vi "Process.vi"(8 "error in (no error)":errorcluster, 10 "Pound in":refnum<class "Pound.lvclass">, 11 "Qbus in":refnum<class "Qbus.lvclass">) -> (0 "error out":errorcluster)   [LabVIEW 2017, in "McsaFpgaBitfileManager.lvlib"]
doc: "Downloads the appropriate bitfile to the device FPGA so that the device can begin to acquire data. The FPGA Acquisition process cannot initiate data acquisition until the device FPGA receives the bitfile."
uses:
  <vilib>/addons/InsightCM/Devices/Shared/Mcsa/McsaFpgaBitfileManager/McsaFpgaBitfileManager.lvlib
  <vilib>/addons/Qbus/Qbus.lvclass
  <vilib>/NI/Software Watchdog/Pound/Pound.lvclass
  <vilib>/addons/InsightCM/Devices/Shared/Mcsa/McsaFpgaBitfileManager/controls/config.ctl
  <vilib>/FPGAPlugInAG/Dynamic/niLvFpga_Close_Dynamic.vi
  <vilib>/rvi/interface/nirviCloseFPGA/nirviCloseFPGA.xnode
  <vilib>/NI/Software Watchdog/Watchdog/Watchdog.lvclass
  <vilib>/addons/InsightCM/Devices/Shared/Common/FpgaBitfileManager/FpgaBitfileManager.lvlib
  <vilib>/addons/InsightCM/Utilities/GlobalConfiguration/GlobalConfiguration.lvlib
  <vilib>/addons/TraceLogger/TraceLogger.lvlib
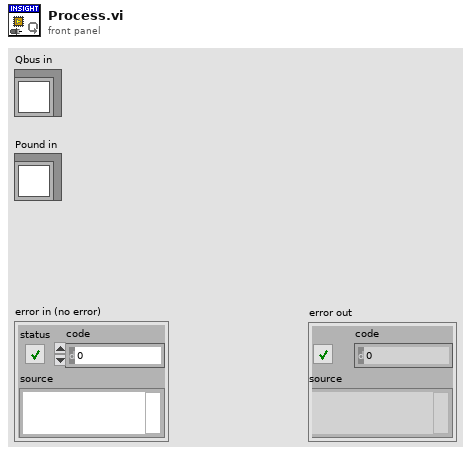
[diagram p1: front panel]
types:
  T1 = typedef "McsaFPGABitfileManager.lvlib/config.ctl" = cluster{"Bitfile reference":refnum<k20>}
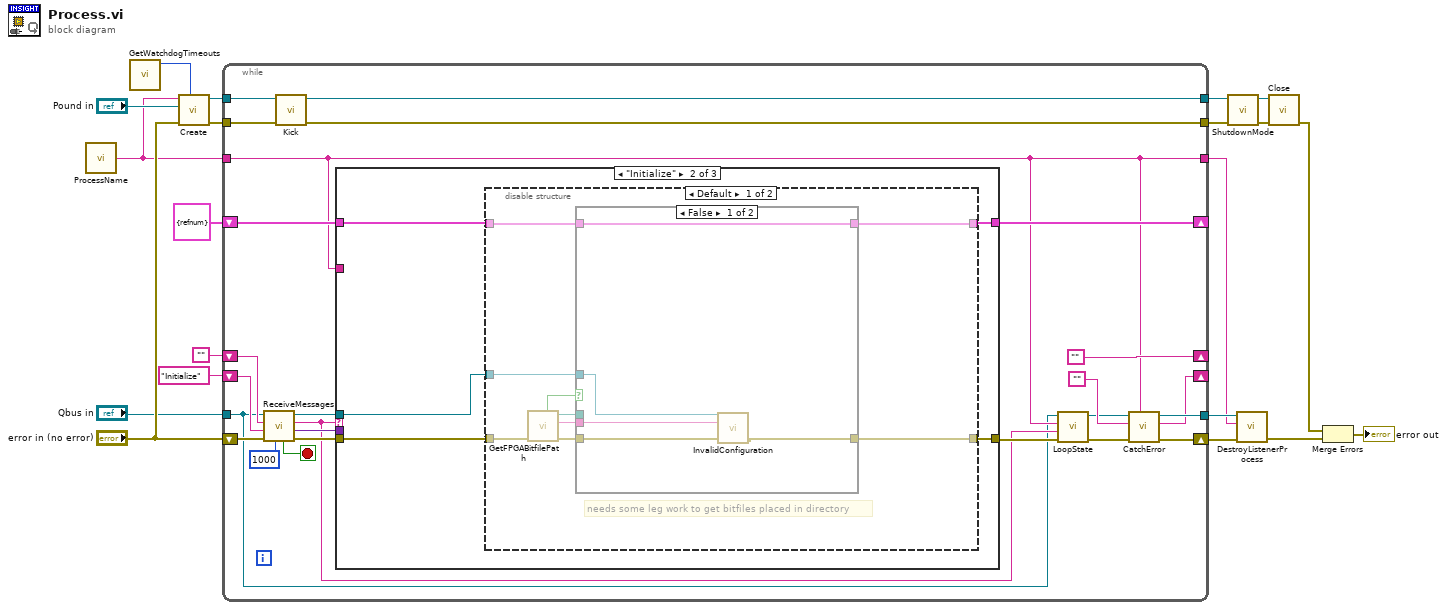
[diagram p0: block diagram]
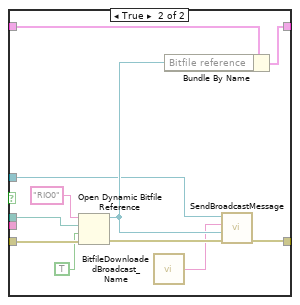
[diagram p3: hidden frame]
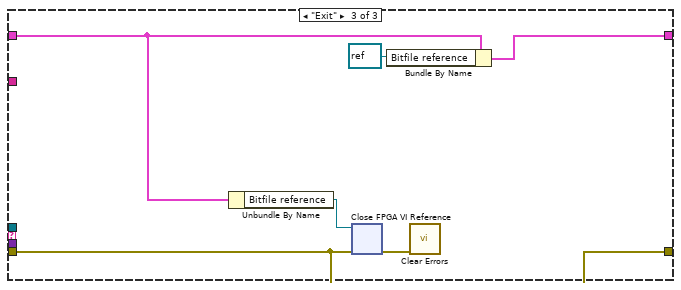
[diagram p5: hidden frame]
diagram:
  n1 = call <vilib>:"ProcessName.vi"() -> ("process name"=w1:string)  [unwired: 5 in]
  n2 = call <vilib>:"GetWatchdogTimeouts.vi"() -> ("software timeout"=w2:u32)  [unwired: 10 in, 1 out]
  n3 = call <vilib>:"Create.vi"("Execution Timeout (ms)"=w2, "error in (no error)"="error in (no error)", "Pound"="Pound in", "Name"=w1) -> ("error out"=w9:errorcluster, "Watchdog"=w14:refnum<data-value>)  [unwired: 6 in]
  n4 = while {
    shift-right: [""] -> _
    shift-left: "" -> [w44]
    tunnel: "Qbus in" -> [w24]
    tunnel: w1 -> [w31]
    tunnel: [w35] -> w18
    tunnel: [w31] -> w17
    shift-right: [w33] -> _
    shift-left: "Initialize" -> [w39]
    shift-right: [w37] -> _
    shift-left: T1 {"Bitfile reference"=refnum} ("config") -> [w38]
    tunnel: w14 -> [w30]
    tunnel: [w29] -> w11
    tunnel: w9 -> [w28]
    tunnel: [w26] -> w8
    shift-right: [w36] -> w19
    shift-left: "error in (no error)" -> [w27]
    stop <- w45 stop-if-true
    n5 = call <vilib>:"ReceiveMessages.vi"("timeout(1000)"=1000 ("Timeout(100)"), "error in (no error)"=w27, "priority action"=w39, "default action"=w44, "Qbus in"=w24) -> ("error out"=w43:errorcluster, "message value"=w40:variant, "action"=w25:string, "Qbus out"=w41:refnum<class "Qbus.lvclass">, "exit"=w45:bool)  [unwired: 2 in]
    n6 = call <vilib>:"Kick.vi"("error in (no error)"=w28, "Watchdog"=w30) -> ("error out"=w26:errorcluster, "Watchdog"=w29:refnum<data-value>)  [unwired: 8 in]
    n7 = case shown="\"Initialize\"" w25 {
      tunnel: w43 -> [w47 w49 w81]
      tunnel: w41 -> [_ w48 _]
      tunnel: [w47 w50 w81] -> w32
      tunnel: w40 -> [_ _ _]
      tunnel: w38 -> [w46 w52 w82]
      tunnel: [w46 w51 w85] -> w37
      tunnel: w31 -> [_ _ _]
      frame "", Default {
      }
      frame "Initialize" {
        n8 = disable-structure shown="Default" {
          disable-tunnel: w49 -> [w61 w78]
          disable-tunnel: w52 -> [w60 w79]
          disable-tunnel: [w59 w79] -> w51
          disable-tunnel: [w58 w78] -> w50
          disable-tunnel: w48 -> [w57 _]
          frame condition #0 {
            # "needs some leg work to get bitfiles placed in directory"
            n9 = call <vilib>:"GetFPGABitfilePath.vi"("error in (no error)"=w61) -> ("error out"=w55:errorcluster, "description"=w54:string, "fpga bitfile"=w56:path, "found"=w53:bool)  [unwired: 7 in]
            n10 = case shown="False" w53 {
              tunnel: w56 -> [_ w77]
              tunnel: w55 -> [w65 w75]
              tunnel: [w64 w69] -> w58
              tunnel: w60 -> [w66 w73]
              tunnel: [w66 w72] -> w59
              tunnel: w57 -> [w63 w68]
              tunnel: w54 -> [w62 _]
              frame False {
                n11 = call <vilib>:"InvalidConfiguration.vi"("error in (no error)"=w65, "description"=w62, "Qbus in"=w63) -> ("error out"=w64:errorcluster)  [unwired: 7 in, 1 out]
              }
              frame True {
                n12 = Open Dynamic Bitfile Reference(0:"RIO0" ("Device address"), 1:w77, 2:TRUE ("Run When Loaded"), 3:w75) -> (5:w71:refnum<k20>, 8:w70:errorcluster)  [unwired: 1 in]
                n13 = call <vilib>:"BitfileDownloadedBroadcast_Name.vi"() -> ("message name"=w67:string)  [unwired: 5 in]
                n14 = Bundle By Name(cluster=w73, "Bitfile reference"=w71) -> (w72:T1)
                n15 = call <vilib>:"SendBroadcastMessage.vi"("error in (no error)"=w70, "message value"=w71, "message name"=w67, "Qbus in"=w68) -> ("error in (no error)"=w69:errorcluster)  [unwired: 6 in, 1 out]
              }
            }
          }
          frame condition #1 (active) {
          }
        }
      }
      frame "Exit" {
        n16 = Unbundle By Name(w82) -> ("Bitfile reference"=w84:refnum<k20>)
        n17 = xnode "Close FPGA VI Reference"("FPGA VI Reference In"=w84, "error in"=w81) -> ("error out"=w80:errorcluster)
        n18 = Bundle By Name(cluster=w82, "Bitfile reference"=refnum<k20> refnum) -> (w85:T1)
        n19 = call <vilib>:"Clear Errors.vi"("error in (no error)"=w80) -> ()  [unwired: 5 in, 2 out]
      }
    }
    n20 = call <vilib>:"LoopState.vi"("error in (no error)"=w32, "loop action"=w25, "process name"=w31, "Qbus in"=w24) -> ("error out"=w22:errorcluster, "Qbus out"=w21:refnum<class "Qbus.lvclass">)  [unwired: 6 in]
    n21 = call <vilib>:"CatchError.vi"("source"=w31, "error in (no error)"=w22, "next action in"="", "Qbus in"=w21) -> ("error out"=w36:errorcluster, "next action out"=w33:string, "Qbus out"=w35:refnum<class "Qbus.lvclass">)  [unwired: 5 in]
  }
  n22 = call <vilib>:"ShutdownMode.vi"("error in (no error)"=w8, "Watchdog"=w11) -> ("error out"=w10:errorcluster, "Watchdog"=w12:refnum<data-value>)  [unwired: 8 in]
  n23 = call <vilib>:"DestroyListenerProcess.vi"("error in (no error)"=w19, "process name"=w17, "Qbus in"=w18) -> ("error in (no error)"=w7:errorcluster)  [unwired: 7 in, 1 out]
  n24 = call <vilib>:"Close.vi"("error in (no error)"=w10, "Watchdog"=w12) -> ("error out"=w6:errorcluster)  [unwired: 9 in]
  n25 = Merge Errors(w6, w7) -> (→"error out":errorcluster)
